vi "mxwScript_API_XMLTemplateName_AddSetDiagram.vi"(8 "error in (no error)":errorcluster, 10 "path":string, 11 "absolutePath":string) -> (0 "error out":errorcluster, 3 "encoded absolutePath":string)   [LabVIEW 2020]
doc: "After dropping the template, set a diagram on the new code as the current diagram. <B>path</B> is the path in the template code to the new diagram."
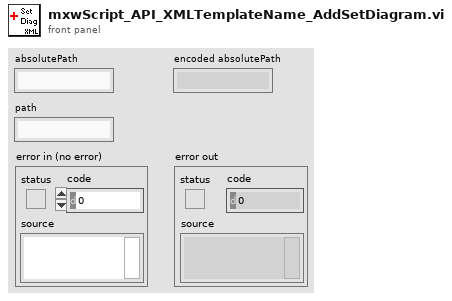
[diagram p1: front panel]
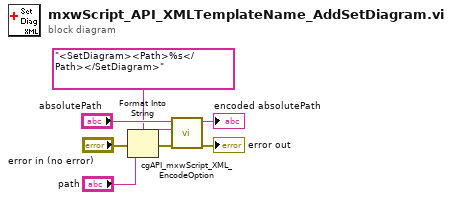
[diagram p0: block diagram]
diagram:
  n1 = Format Into String(format string="<SetDiagram><Path>%s</Path></SetDiagram>" ("control name"), error in="error in (no error)", "path") -> (resulting string=w2:string, error out=w4:errorcluster)  [unwired: 1 in]
  n2 = call "cgAPI_mxwScript_XML_EncodeOption.vi"("error in (no error)"=w4, "otherXML"=w2, "normalTextString"="absolutePath") -> ("error out"=→"error out":errorcluster, "encodedString"=→"encoded absolutePath":string)  [unwired: 7 out]
